vi "SendToRecord (Path).vi"(8 "error in (no error)":errorcluster, 10 "Path":path, 11 "Qbus in":refnum<class "Qbus.lvclass">) -> (0 "error out":errorcluster)   [LabVIEW 2015, in "FileHandler.lvlib"]
uses:
  FileHandler.lvlib
  <vilib>/addons/Qbus/Qbus.lvclass
  controls/Record.ctl
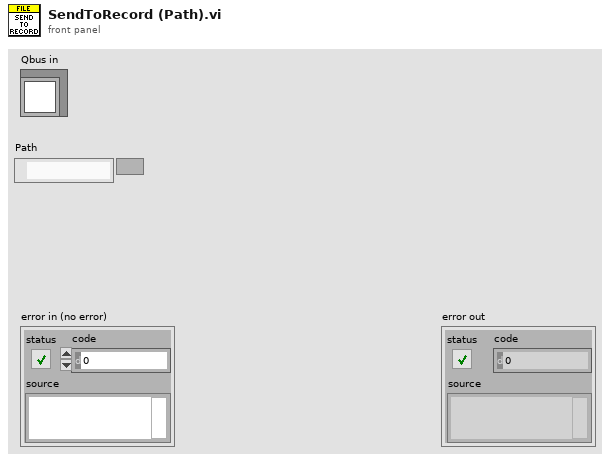
[diagram p1: front panel]
types:
  T1 = typedef "FileHandler.lvlib/Record.ctl" = cluster{"Time":timestamp, "Path":path}
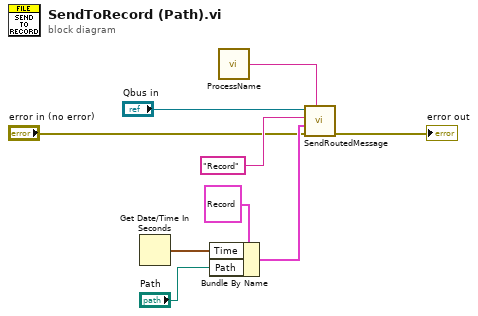
[diagram p0: block diagram]
diagram:
  n1 = Get Date/Time In Seconds() -> (seconds since 1Jan1904=w4:timestamp)
  n2 = Bundle By Name(cluster=T1 {"Time"=timestamp(0 s since 1904-01-01), "Path"=path ""} ("Record"), "Time"=w4, "Path"="Path") -> (w5:T1)
  n3 = call "ProcessName.vi"() -> ("process name"=w9:string)  [unwired: 5 in]
  n4 = call <vilib>:"SendRoutedMessage.vi"("listener process"=w9, "error in (no error)"="error in (no error)", "message value"=w5, "message name"="Record", "Qbus in"="Qbus in") -> ("error in (no error)"=→"error out":errorcluster)  [unwired: 5 in, 1 out]
